vi "Coordenadas_Str_a_Coordenadas_Int.vi"(3 "Coordenadas_Str":string) -> (0 "Columna":i32, 1 "Fila":i32)   [LabVIEW 2019]
doc: "Separa la cadena con coordenadas 'x,y' a coordenadas 'x' e 'y' de tipo entero."
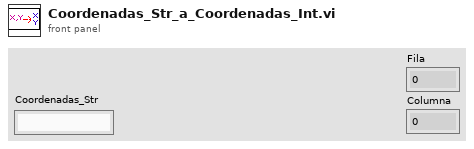
[diagram p1: front panel]
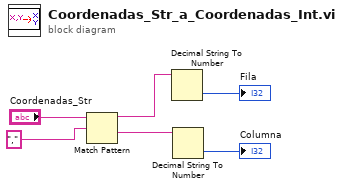
[diagram p0: block diagram]
diagram:
  n1 = Match Pattern(string="Coordenadas_Str", regular expression=",") -> (before substring=w4:string, after substring=w3:string)  [unwired: 1 in, 2 out]
  n2 = Decimal String To Number(string=w4) -> (number=→"Fila":i32)  [unwired: 2 in, 1 out]
  n3 = Decimal String To Number(string=w3) -> (number=→"Columna":i32)  [unwired: 2 in, 1 out]
